vi "Calculate F(x).vi"() -> (2 "val1":dbl, 3 "f(x)":dbl)   [LabVIEW 2020]
panel:
  out "Waveform Graph 2":dbl[](graph)
  out "Waveform Graph":dbl[](graph)
  out "Output Array":dbl[][](array[numeric])
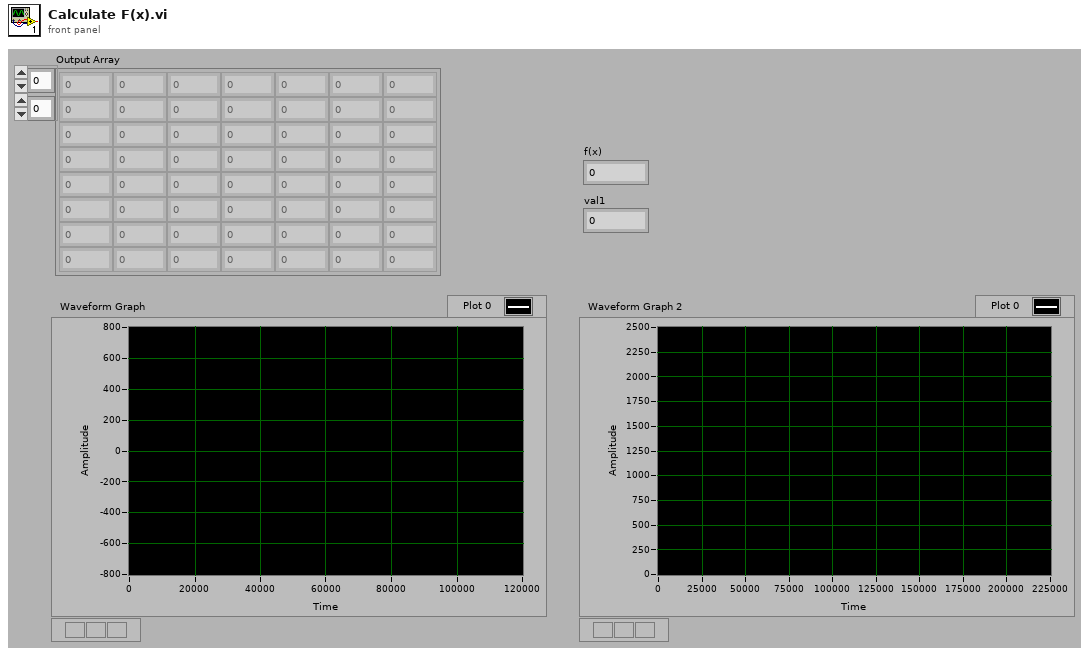
[diagram p1: front panel]
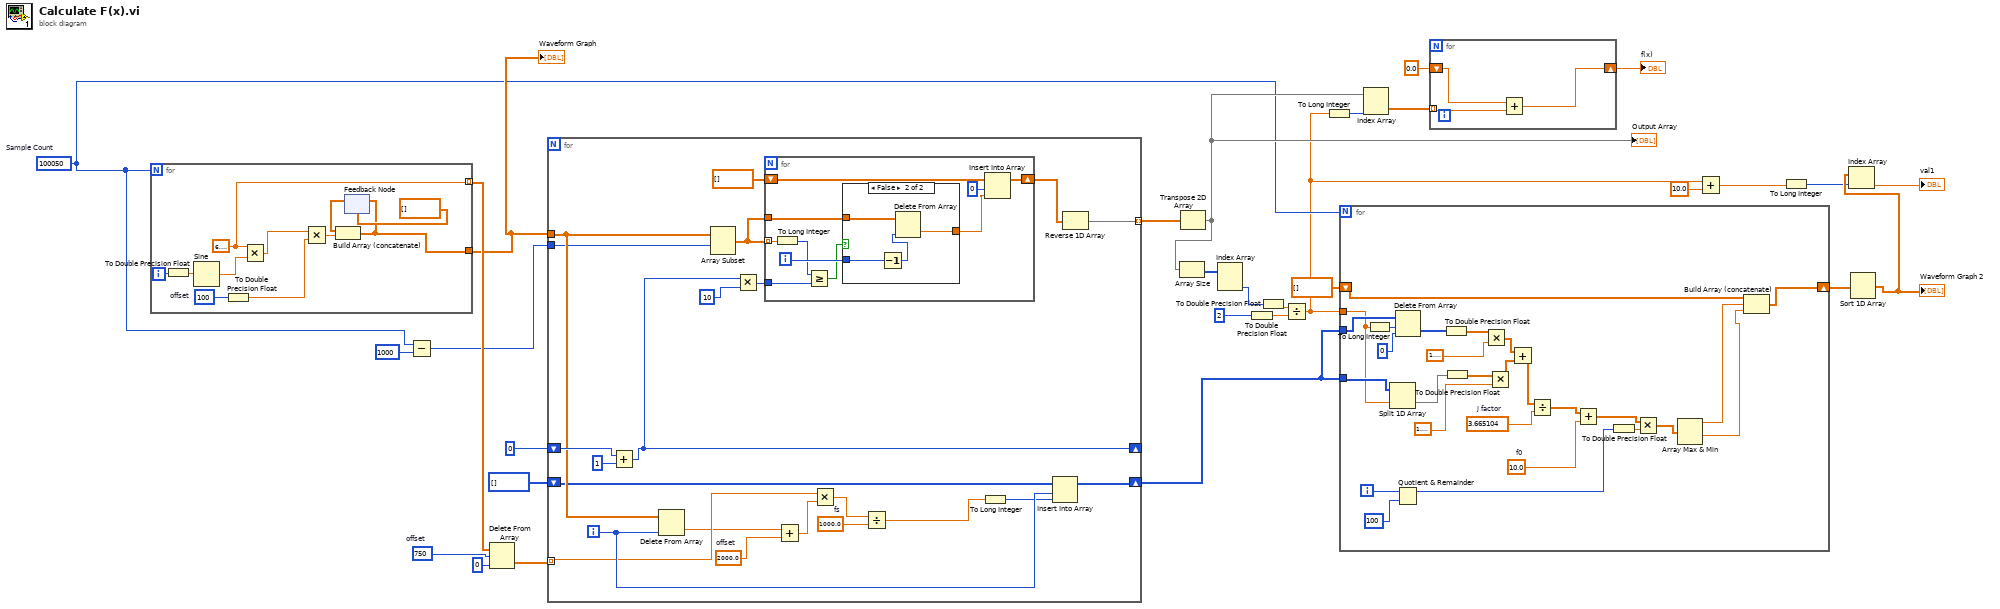
[diagram p0: block diagram]
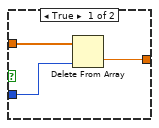
[diagram p2: hidden frame]
diagram:
  w11 = 100050  # Sample Count
  w13 = 750  # offset
  n1 = for {
    N: w11 -> [_]
    tunnel: [w36] -> w27 mode=indexing
    tunnel: [w33] -> w12
    i -> [w38]
    w35 = 100  # offset
    w36 = 6.283185307179586
    n2 = To Double Precision Float(number=w38) -> (double precision float=w37:dbl)
    n3 = Sine(x=w37) -> (sin(x)=w41:dbl)
    n4 = To Double Precision Float(number=w35) -> (double precision float=w34:dbl)
    n5 = Multiply(x=w36, y=w41) -> (x*y=w40:dbl)
    n6 = Multiply(x=w40, y=w34) -> (x*y=w32:dbl)
    n7 = feedback #1(dbl[] []) -> (w31:dbl[])
    n8 = Build Array (concatenate)(w31, w32) -> (w33:dbl[])
    n9 = feedback-in #1(w33) -> ()
  }
  "Waveform Graph" <- w12
  n10 = Subtract(x=w11, y=1000) -> (x-y=w16:i32)
  n11 = Delete From Array(array=w27, length=w13, index=0) -> (deleted portion=w14:dbl[])  [unwired: 1 out]
  n12 = for {
    tunnel: w12 -> [w54]
    tunnel: w16 -> [w49]
    tunnel: [w60] -> w30 mode=indexing
    shift-right: [w57] -> _
    shift-left: 0 -> [w58]
    shift-right: [w52] -> w25
    shift-left: i32[] [] -> [w53]
    tunnel: w14 -> [w50] mode=indexing
    i -> [w51]
    w42 = 1000.0  # fs
    w45 = 2000.0  # offset
    n13 = Add(x=w58, y=1) -> (x+y=w57:i32)
    n14 = Delete From Array(array=w54, index=w51) -> (deleted portion=w48:dbl)  [unwired: 1 in, 1 out]
    n15 = Array Subset(array=w54, index=w49) -> (w63:dbl[])  [unwired: 1 in]
    n16 = Multiply(x=w57, y=10) -> (x*y=w55:i32)
    n17 = for {
      tunnel: w63 -> [w73] mode=indexing
      tunnel: w63 -> [w69]
      shift-right: [w71] -> w61
      shift-left: dbl[] [] ("array") -> [w72]
      tunnel: w55 -> [w70]
      i -> [w68]
      n18 = To Long Integer(number=w73) -> (32bit integer=w64:i32)
      n19 = Greater Or Equal?(x=w64, y=w70) -> (x >= y?=w65:bool)
      n20 = case shown="False" w65 {
        tunnel: w69 -> [w76 w80]
        tunnel: w68 -> [w75 w77]
        tunnel: [w74 w79] -> w66
        frame True {
          n21 = Delete From Array(array=w76, index=w75) -> (deleted portion=w74:dbl)  [unwired: 1 in, 1 out]
        }
        frame False {
          n22 = Decrement(x=w77) -> (x-1=w78:i32)
          n23 = Delete From Array(array=w80, index=w78) -> (deleted portion=w79:dbl)  [unwired: 1 in, 1 out]
        }
      }
      n24 = Insert Into Array(array=w72, index=0, new element=w66) -> (w71:dbl[])
    }
    n25 = Add(x=w48, y=w45) -> (x+y=w44:dbl)
    n26 = Multiply(x=w50, y=w44) -> (x*y=w43:dbl)
    n27 = Divide(x=w43, y=w42) -> (x/y=w47:dbl)
    n28 = To Long Integer(number=w47) -> (32bit integer=w46:i32)
    n29 = Insert Into Array(array=w53, index=w51, new element=w46) -> (w52:i32[])
    n30 = Reverse 1D Array(array=w61) -> (reversed array=w60:dbl[])
  }
  n31 = Transpose 2D Array(2D array=w30) -> (transposed array=w21:dbl[][])
  "Output Array" <- w21
  n32 = Array Size(array=w21) -> (size(s)=w26:i32[])
  n33 = Index Array(array=w26) -> (element #2=w6:i32)  [unwired: 2 in, 1 out]
  n34 = To Double Precision Float(number=2 ("y")) -> (double precision float=w8:dbl)
  n35 = To Double Precision Float(number=w6) -> (double precision float=w7:dbl)
  n36 = Divide(x=w7, y=w8) -> (x/y=w4:dbl)
  n37 = To Long Integer(number=w4) -> (32bit integer=w5:i32)
  n38 = for {
    N: w11 -> [_]
    tunnel: w25 -> [w107]
    tunnel: w4 -> [w85]
    tunnel: w25 -> [w103]
    shift-right: [w91] -> w10
    shift-left: dbl[] [] -> [w98]
    i -> [w102]
    w104 = 10.0  # f0
    w106 = 3.665104  # j factor
    n39 = To Long Integer(number=w85) -> (32bit integer=w86:i32)
    n40 = Split 1D Array(array=w107, index=w85) -> (second subarray=w84:i32[])  [unwired: 1 out]
    n41 = Delete From Array(array=w103, length=w86, index=0) -> (deleted portion=w87:i32[])  [unwired: 1 out]
    n42 = Quotient & Remainder(x=w102, y=100) -> (x-y*floor(x/y)=w82:i32)  [unwired: 1 out]
    n43 = To Double Precision Float(number=w87) -> (double precision float=w88:dbl[])
    n44 = To Double Precision Float(number=w84) -> (double precision float=w83:dbl[])
    n45 = Multiply(x=w88, y=1.5707963267948966) -> (x*y=w94:dbl[])
    n46 = Multiply(x=w83, y=1.5707963267948966) -> (x*y=w93:dbl[])
    n47 = Add(x=w94, y=w93) -> (x+y=w92:dbl[])
    n48 = Divide(x=w92, y=w106) -> (x/y=w105:dbl[])
    n49 = Add(x=w105, y=w104) -> (x+y=w100:dbl[])
    n50 = To Double Precision Float(number=w82) -> (double precision float=w81:dbl)
    n51 = Multiply(x=w100, y=w81) -> (x*y=w99:dbl[])
    n52 = Array Max & Min(array=w99) -> (max value=w90:dbl, min value=w89:dbl)  [unwired: 2 out]
    n53 = Build Array (concatenate)(w98, w90, w89) -> (w91:dbl[])
  }
  n54 = Index Array(array=w21, index (col)=w5) -> (element=w20:dbl[])  [unwired: 1 in]
  n55 = for {
    tunnel: w20 -> [w110] mode=indexing
    shift-right: [w108] -> w18
    shift-left: 0.0 ("x") -> [w109]
    n56 = Add(x=w109, y=w110) -> (x+y=w108:dbl)
  }
  "f(x)" <- w18
  n57 = Add(x=w4, y=10.0) -> (x+y=w2:dbl)
  n58 = To Long Integer(number=w2) -> (32bit integer=w1:i32)
  n59 = Sort 1D Array(array=w10) -> (sorted array=w3:dbl[])
  "Waveform Graph 2" <- w3
  n60 = Index Array(array=w3, index=w1) -> (element=→"val1":dbl)
